vi "niFPGA I32xI32 MAC - FXP.vi"(5 "A":i32 format="%.0x", 7 "B":i32 format="%.0x", 9 "C":fxp<+/-,36,32> format="%.0x") -> (8 "A*B+C":fxp<+/-,36,32>=2838.0 format="%.14g")   [LabVIEW 2017]
doc: "This utility VI implements a 32 x 32 multiply and accumulate that returns a signed <36,32> FXP result. It requires four 16 x 16 = 32 multipliers to compute the partial products, and adds in the accumulate value in parallel with the partial product adds to improve timing performance. \n\nThe VI is similar in functionality to niFPGA I32xI32 MAC+ MSB.vi, but returns 4 extra LSBs for increased accuracy. \n\nThe output rounding mode is round-half-up, and is achieved at no extra cost by incorporating the rounding bit into the accumulate add. \n\nThis VI does not handle overflow; it assumes the inputs are constrained to prevent overflow."
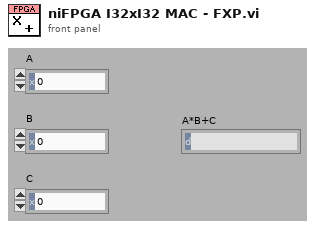
[diagram p1: front panel]
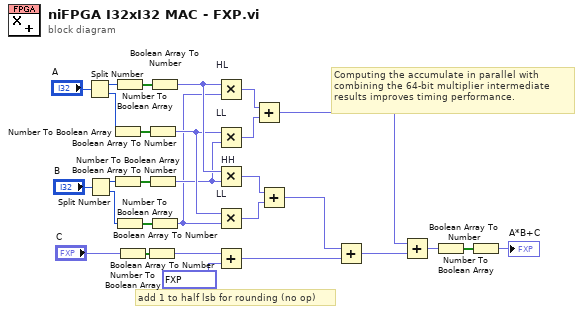
[diagram p0: block diagram]
diagram:
  # "add 1 to half lsb for rounding (no op)"
  # "Computing the accumulate in parallel with \ncombining the 64-bit multiplier intermediate \nresults improves timing performance."
  n1 = Split Number(x="A") -> (hi(x)=w29:u16, lo(x)=w15:u16)
  n2 = Split Number(x="B") -> (hi(x)=w17:u16, lo(x)=w13:u16)
  n3 = Number To Boolean Array(number=w15) -> (Boolean array=w16:bool[])
  n4 = Number To Boolean Array(number=w17) -> (Boolean array=w18:bool[])
  n5 = Number To Boolean Array(number=w29) -> (Boolean array=w20:bool[])
  n6 = Number To Boolean Array(number=w13) -> (Boolean array=w14:bool[])
  n7 = Number To Boolean Array(number="C") -> (Boolean array=w21:bool[])
  n8 = Boolean Array To Number(Boolean array=w21) -> (number=w9:fxp<+/-,36,0>)
  n9 = Boolean Array To Number(Boolean array=w16) -> (number=w6:fxp<+,16,-16>)
  n10 = Boolean Array To Number(Boolean array=w18) -> (number=w4:fxp<+/-,16,0>)
  n11 = Boolean Array To Number(Boolean array=w20) -> (number=w19:fxp<+/-,16,0>)
  n12 = Boolean Array To Number(Boolean array=w14) -> (number=w3:fxp<+,16,-16>)
  n13 = Multiply "HL"(x=w19, y=w3) -> (x*y=w11:fxp<+/-,32,-16>)
  n14 = Multiply "LL"(x=w6, y=w4) -> (x*y=w12:fxp<+/-,32,-16>)
  n15 = Multiply "HH"(x=w19, y=w4) -> (x*y=w27:fxp<+/-,32,0>)
  n16 = Multiply "LL"(x=w6, y=w3) -> (x*y=w26:fxp<+,32,-32>)
  n17 = Add(x=w9, y=fxp<+,1,-36> 7.275957614183426e-12) -> (x+y=w7:fxp<+/-,37,0>)
  n18 = Add(x=w11, y=w12) -> (x+y=w1:fxp<+/-,33,-15>)
  n19 = Add(x=w27, y=w26) -> (x+y=w2:fxp<+/-,64,0>)
  n20 = Add(x=w2, y=w7) -> (x+y=w28:fxp<+/-,48,0>)
  n21 = Add(x=w1, y=w28) -> (x+y=w5:fxp<+/-,36,0>)
  n22 = Number To Boolean Array(number=w5) -> (Boolean array=w23:bool[])
  n23 = Boolean Array To Number(Boolean array=w23) -> (number=→"A*B+C":fxp<+/-,36,32>)
